vi "ComPortDialog_VISA.vi"(10 "Com-Einst. in":T1={"Baudrate"=enum."9600", "Echo"=TRUE, "Timeout"=200, "VISA"="COM1"}, 11 "ini-File":path) -> (1 "Abbruch":bool, 2 "Com-Einst. out":T1={"Baudrate"=enum."115200", "Echo"=FALSE, "Timeout"=200, "VISA"="COM1"})   [LabVIEW 2012]
uses:
  <vilib>/Utility/config.llb/Read Key (Boolean).vi
  <vilib>/Utility/config.llb/Read Key (String).vi
  <vilib>/Utility/config.llb/Read Key (U32).vi
  <vilib>/Utility/config.llb/Write Key (Boolean).vi
  <vilib>/Utility/config.llb/Write Key (String).vi
  <vilib>/Utility/config.llb/Write Key (I32).vi
  <vilib>/Utility/config.llb/Write Key (U32).vi
  <vilib>/Utility/config.llb/NI_LVConfig.lvlib
panel:
  in  "VISA":refnum<visa-resource-name>="COM1"
  in  "Echo":bool
  out "error out":errorcluster caption="Fehler (Ausgang)"
  in  "Baudrate":enum16{"9600", "115200"}(ring)=enum."115200"
  in  "Timeout":u32=100
  in  "cancel":bool
  in  "ok":bool
  in  "Enum":enum16{"wahl", "openCom", "weiter"}(ring)
  in  "error in (no error)":errorcluster caption="Fehler (Eingang - kein Fehler)"
  # "Open ComPort"
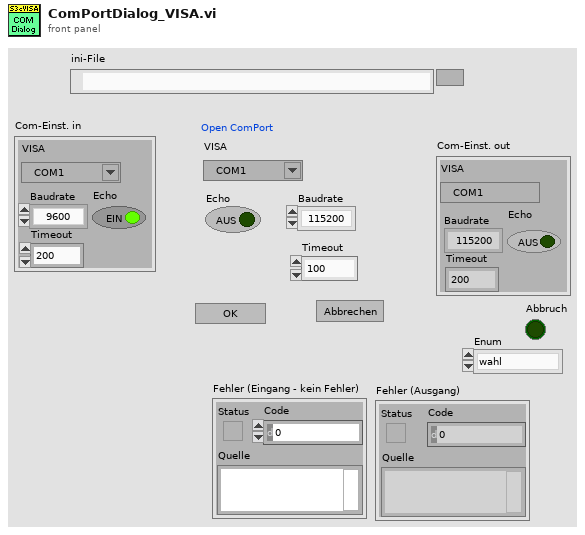
[diagram p1: front panel]
types:
  T1 = cluster{"Baudrate":enum16{"9600", "115200"}, "Echo":bool, "Timeout":u32, "VISA":refnum<visa-resource-name>}
  T2 = typedef "NI_LVConfig.lvlib/Config Data RefNum.ctl" = refnum<k1>
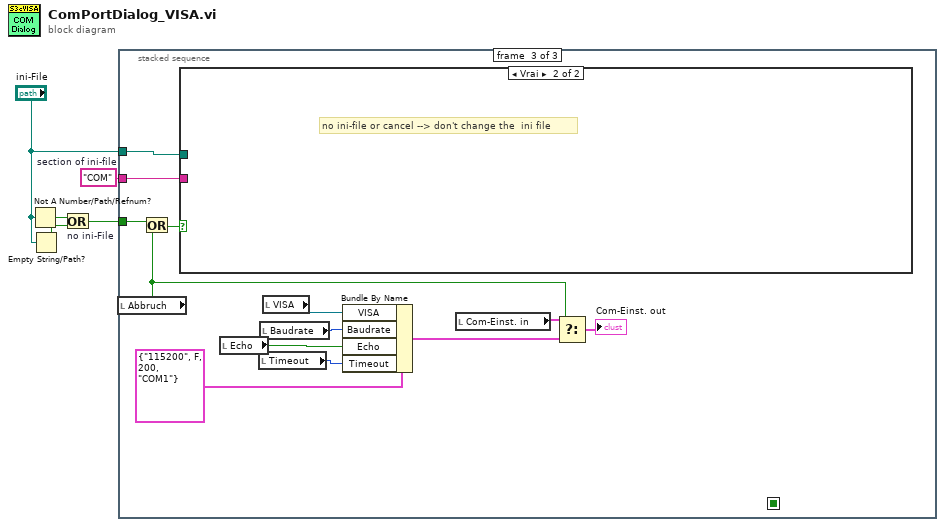
[diagram p0: block diagram]
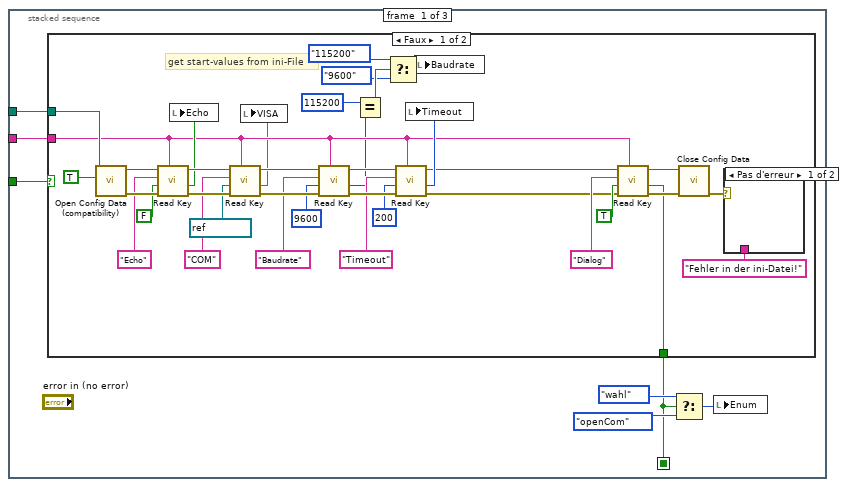
[diagram p2: hidden frame]
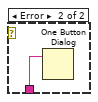
[diagram p3: hidden frame]
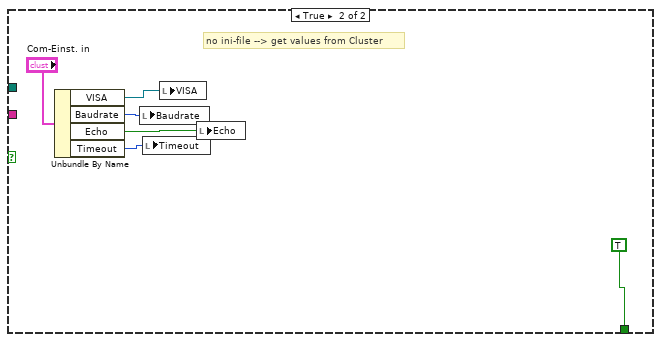
[diagram p4: hidden frame]
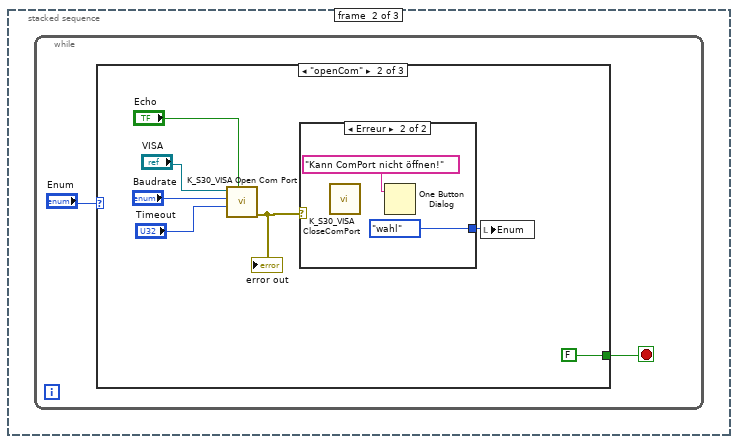
[diagram p5: hidden frame]
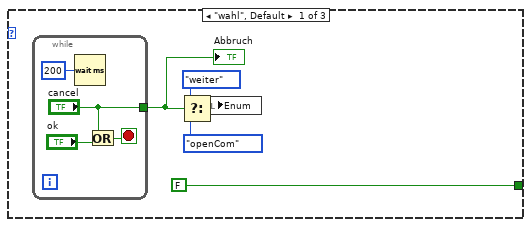
[diagram p6: hidden frame]
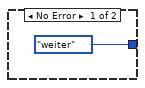
[diagram p7: hidden frame]
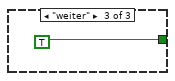
[diagram p8: hidden frame]
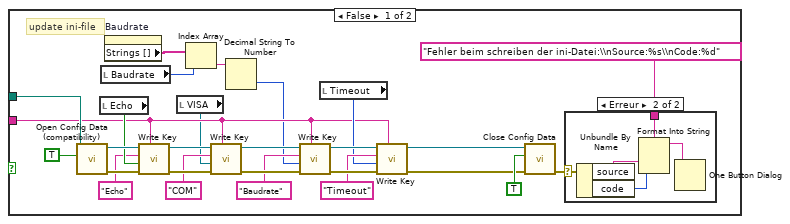
[diagram p9: hidden frame]
diagram:
  w1 = "COM"  # section of ini-file
  n1 = Not A Number/Path/Refnum?(number/path/refnum="ini-File") -> (NaN/Path/Refnum?=w5:bool)
  n2 = Empty String/Path?(string/path="ini-File") -> (empty?=w4:bool)
  n3 = Or "no ini-File"(x=w5, y=w4) -> (x .or. y?=w3:bool)
  n4 = stacked-sequence {
    seq-local: [w7 _ _] -> [_ _ _]
    tunnel: w3 -> [w12 _ w91]
    tunnel: "ini-File" -> [w11 _ w89]
    tunnel: w1 -> [w6 _ w80]
    frame #0 {
      n5 = case shown="Faux" w12 {
        tunnel: w11 -> [w49 _]
        tunnel: [w25 TRUE ("value")] -> w7
        tunnel: w6 -> [w22 _]
        frame False {
          # "get start-values from ini-File"
          n6 = call <vilib>:"Open Config Data (compatibility).vi"("create file if necessary (T)"=TRUE ("create file if necessary? (T)"), "configuration file path"=w49) -> ("error out"=w43:errorcluster, "refnum"=w47:T2)  [unwired: 7 in, 1 out]
          n7 = call-poly <vilib>:"Read Key.vi"("section"=w22, "error in (no error)"=w43, "default value"=FALSE, "key"="Echo", "refnum"=w47) -> ("error out"=w42:errorcluster, "value"=w37:bool, "refnum out"=w46:T2)  [unwired: 3 in, 1 out]
          n8 = local write "Echo"(w37) -> ()
          n9 = call-poly <vilib>:"Read Key.vi"("section"=w22, "error in (no error)"=w42, "default value"=refnum<visa-resource-name> "COM1" ("VISA"), "key"="COM", "refnum"=w46) -> ("error out"=w41:errorcluster, "value"=w13:string, "refnum out"=w45:T2)  [unwired: 3 in, 1 out]
          n10 = local write "VISA"(w13) -> ()
          n11 = call-poly <vilib>:"Read Key.vi"("section"=w22, "error in (no error)"=w41, "default value"=u32 9600, "key"="Baudrate", "refnum"=w45) -> ("error out"=w40:errorcluster, "value"=w20:u32, "refnum out"=w44:T2)  [unwired: 3 in, 1 out]
          n12 = Equal?(x=u32 115200, y=w20) -> (x = y?=w18:bool)
          n13 = Select(t=enum16{"9600", "115200"}."115200", s=w18, f=enum16{"9600", "115200"}."9600") -> (s? t:f=w15:enum16{"9600", "115200"})
          n14 = call-poly <vilib>:"Read Key.vi"("section"=w22, "error in (no error)"=w40, "default value"=u32 200, "key"="Timeout", "refnum"=w44) -> ("error out"=w24:errorcluster, "value"=w30:u32, "refnum out"=w23:T2)  [unwired: 3 in, 1 out]
          n15 = local write "Timeout"(w30) -> ()
          n16 = local write "Baudrate"(w15) -> ()
          n17 = call-poly <vilib>:"Read Key.vi"("section"=w22, "error in (no error)"=w24, "default value"=TRUE, "key"="Dialog", "refnum"=w23) -> ("error out"=w27:errorcluster, "value"=w25:bool, "refnum out"=w26:T2)  [unwired: 3 in, 1 out]
          n18 = call <vilib>:"Close Config Data.vi"("error in (no error)"=w27, "refnum"=w26) -> ("error out"=w32:errorcluster)  [unwired: 8 in, 1 out]
          n19 = case shown="Pas d'erreur" w32 {
            tunnel: "Fehler in der ini-Datei!" ("Nachricht") -> [_ w50]
            frame No Error {
            }
            frame Error {
              n20 = One Button Dialog(message=w50) -> ()  [unwired: 1 in, 1 out]
            }
          }
        }
        frame True {
          # "no ini-file --> get values from Cluster"
          n21 = Unbundle By Name("Com-Einst. in") -> ("VISA"=w51:refnum<visa-resource-name>, "Baudrate"=w55:enum16{"9600", "115200"}, "Echo"=w53:bool, "Timeout"=w54:u32)
          n22 = local write "Baudrate"(w55) -> ()
          n23 = local write "Timeout"(w54) -> ()
          n24 = local write "VISA"(w51) -> ()
          n25 = local write "Echo"(w53) -> ()
        }
      }
      n26 = Select(t=enum16{"wahl", "openCom", "weiter"}."wahl" ("Enum"), s=w7, f=enum16{"wahl", "openCom", "weiter"}."openCom" ("Enum")) -> (s? t:f=w10:enum16{"wahl", "openCom", "weiter"})
      n27 = local write "Enum"(w10) -> ()
    }
    frame #1 {
      n28 = while {
        stop <- w57 stop-if-true
        n29 = case shown="\"openCom\"" "Enum" {
          tunnel: [FALSE FALSE TRUE] -> w57
          frame "wahl", Default {
            n30 = while {
              tunnel: ["cancel"] -> w62
              stop <- w66 stop-if-true
              n31 = Wait (ms)(milliseconds to wait=u32 200 ("Zu wartende ms")) -> ()  [unwired: 1 out]
              n32 = Or(x="cancel", y="ok") -> (x .or. y?=w66:bool)
            }
            "Abbruch" <- w62
            n33 = Select(t=enum16{"wahl", "openCom", "weiter"}."weiter" ("Enum"), s=w62, f=enum16{"wahl", "openCom", "weiter"}."openCom" ("Enum")) -> (s? t:f=w61:enum16{"wahl", "openCom", "weiter"})
            n34 = local write "Enum"(w61) -> ()
          }
          frame "openCom" {
            n35 = call "K_S30_VISA Open Com Port.vi"("RS-converter:\necho"="Echo", "timeout"="Timeout", "Baudrate"="Baudrate", "VISA resource name"="VISA") -> ("error out"=w69:errorcluster)  [unwired: 4 in, 1 out]
            "error out" <- w69
            n36 = case shown="Erreur" w69 {
              tunnel: [enum16{"wahl", "openCom", "weiter"}."weiter" ("Enum") enum16{"wahl", "openCom", "weiter"}."wahl" ("Enum")] -> w74
              frame No Error {
              }
              frame Error {
                n37 = call "K_S30_VISA CloseComPort.vi"() -> ()  [unwired: 7 in, 1 out]
                n38 = One Button Dialog(message="Kann ComPort nicht öffnen!" ("Nachricht")) -> ()  [unwired: 1 in, 1 out]
              }
            }
            n39 = local write "Enum"(w74) -> ()
          }
          frame "weiter" {
          }
        }
      }
    }
    frame #2 {
      n40 = local read "Abbruch"() -> (w88:bool)
      n41 = Or(x=w91, y=w88) -> (x .or. y?=w90:bool)
      n42 = case shown="Vrai" w90 {
        tunnel: w89 -> [w102 _]
        tunnel: w80 -> [w97 _]
        frame False {
          # "update ini-file"
          n43 = call <vilib>:"Open Config Data (compatibility).vi"("create file if necessary (T)"=TRUE ("create file if necessary? (T)"), "configuration file path"=w102) -> ("error out"=w113:errorcluster, "refnum"=w117:T2)  [unwired: 7 in, 1 out]
          n44 = local read "Echo"() -> (w109:bool)
          n45 = local read "Baudrate"() -> (w93:enum16{"9600", "115200"})
          n46 = property on="Baudrate" class="Énum (strict)"() -> ("Strings []"=w94:string[])  [unwired: 2 in, 2 out]
          n47 = call-poly <vilib>:"Write Key.vi"("section"=w97, "error in (no error)"=w113, "value"=w109, "key"="Echo", "refnum"=w117) -> ("error out"=w112:errorcluster, "refnum out"=w116:T2)  [unwired: 4 in, 1 out]
          n48 = local read "VISA"() -> (w96:refnum<visa-resource-name>)
          n49 = Index Array(array=w94, index=w93) -> (element=w95:string)
          n50 = call-poly <vilib>:"Write Key.vi"("section"=w97, "error in (no error)"=w112, "value"=w96, "key"="COM", "refnum"=w116) -> ("error out"=w111:errorcluster, "refnum out"=w115:T2)  [unwired: 4 in, 1 out]
          n51 = Decimal String To Number(string=w95) -> (number=w92:i32)  [unwired: 2 in, 1 out]
          n52 = call-poly <vilib>:"Write Key.vi"("section"=w97, "error in (no error)"=w111, "value"=w92, "key"="Baudrate", "refnum"=w115) -> ("error out"=w110:errorcluster, "refnum out"=w114:T2)  [unwired: 4 in, 1 out]
          n53 = local read "Timeout"() -> (w100:u32)
          n54 = call-poly <vilib>:"Write Key.vi"("section"=w97, "error in (no error)"=w110, "value"=w100, "key"="Timeout", "refnum"=w114) -> ("error out"=w99:errorcluster, "refnum out"=w98:T2)  [unwired: 4 in, 1 out]
          n55 = call <vilib>:"Close Config Data.vi"("error in (no error)"=w99, "write file if changed (T)"=TRUE ("write configuration file? (T)"), "refnum"=w98) -> ("error out"=w104:errorcluster)  [unwired: 7 in, 1 out]
          n56 = case shown="Erreur" w104 {
            selector: w104 -> [_ w123]
            tunnel: "Fehler beim schreiben der ini-Datei:\\nSource:%s\\nCode:%d" ("Nachricht") -> [_ w122]
            frame No Error {
            }
            frame Error {
              n57 = Unbundle By Name(w123) -> ("source"=w121:string, "code"=w120:i32)
              n58 = Format Into String(format string=w122, w121, w120) -> (resulting string=w119:string)  [unwired: 2 in, 1 out]
              n59 = One Button Dialog(message=w119) -> ()  [unwired: 1 in, 1 out]
            }
          }
        }
        frame True {
          # "no ini-file or cancel --> don't change the  ini file"
        }
      }
      n60 = local read "Echo"() -> (w83:bool)
      n61 = local read "Timeout"() -> (w82:u32)
      n62 = local read "Baudrate"() -> (w84:enum16{"9600", "115200"})
      n63 = local read "VISA"() -> (w79:refnum<visa-resource-name>)
      n64 = Bundle By Name(cluster=T1 {"Baudrate"=enum."115200", "Echo"=FALSE, "Timeout"=200, "VISA"="COM1"} ("Com-Einst. out"), "VISA"=w79, "Baudrate"=w84, "Echo"=w83, "Timeout"=w82) -> (w81:T1)
      n65 = local read "Com-Einst. in"() -> (w86:T1)
      n66 = Select(t=w86, s=w88, f=w81) -> (s? t:f=→"Com-Einst. out":T1)
    }
  }
